vi "Main.vi"() -> ()   [LabVIEW 2018]
panel:
  in  "退出":bool
  in  "接收":bool
  in  "发送":bool
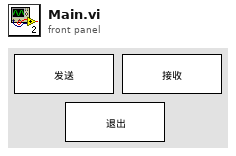
[diagram p1: front panel]
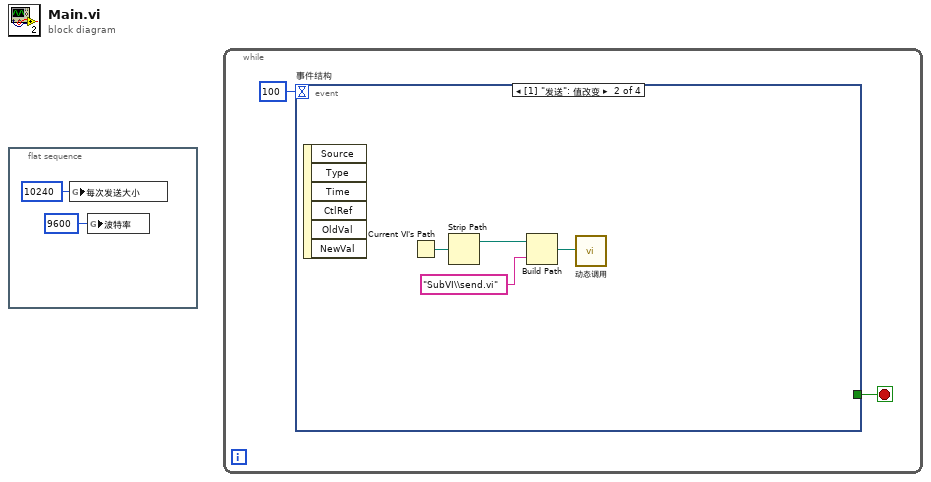
[diagram p0: block diagram]
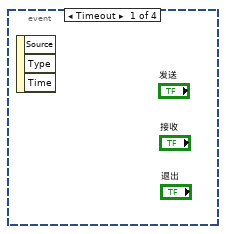
[diagram p2: hidden frame]
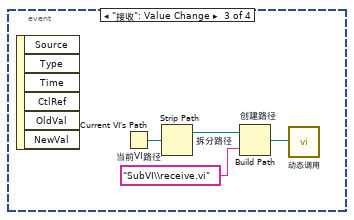
[diagram p3: hidden frame]
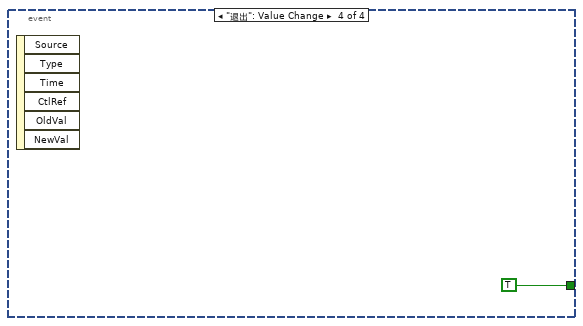
[diagram p4: hidden frame]
diagram:
  n1 = flat-sequence {
    frame #0 {
      n2 = global write "全局变量.vi" "每次发送大小"(10240 ("每次发送大小")) -> ()
      n3 = global write "全局变量.vi" "波特率"(u32 9600 ("波特率")) -> ()
    }
  }
  n4 = while {
    stop <- w3 stop-if-true
    n5 = event "事件结构" shown="[1] \"发送\": 值改变" {
      selector: _ -> [_ _ _ _]
      dyn-events: _ -> [_ _ _ _]
      timeout: 100 -> [_ _ _ _]
      tunnel: [_ _ _ TRUE] -> w3
      event Timeout {
        n6 = event-data() -> ()  [unwired: 1 in, 3 out]
      }
      event "发送": Value Change {
        n7 = event-data() -> ()  [unwired: 1 in, 6 out]
        n8 = Current VI's Path() -> (path=w8:path)
        n9 = Strip Path(path=w8) -> (stripped path=w7:path)  [unwired: 1 out]
        n10 = Build Path(base path=w7, name or relative path="SubVI\\send.vi" ("名称或相对路径")) -> (appended path=w5:path)
        n11 = call "动态调用.vi"("VI路径"=w5) -> ()  [unwired: 11 in]
      }
      event "接收": Value Change {
        n12 = event-data() -> ()  [unwired: 1 in, 6 out]
        n13 = Current VI's Path "当前VI路径"() -> (path=w12:path)
        n14 = Strip Path "拆分路径"(path=w12) -> (stripped path=w11:path)  [unwired: 1 out]
        n15 = Build Path "创建路径"(base path=w11, name or relative path="SubVI\\receive.vi" ("名称或相对路径")) -> (appended path=w9:path)
        n16 = call "动态调用.vi"("VI路径"=w9) -> ()  [unwired: 11 in]
      }
      event "退出": Value Change {
        n17 = event-data() -> ()  [unwired: 1 in, 6 out]
      }
    }
  }
